vi "Bodies_GetPtInXYZ0.vi"(8 "error in (no error)":errorcluster, 10 "Point":T1, 11 "Bodies.lvclass":refnum<class "Bodies.lvclass">) -> (0 "error out":errorcluster, 1 "Coord4InGCS":T1={"Coord4"=[0.0, 0.0, 0.0, 1.0], "ID"=0}, 2 "PointInGCS":dbl[](array[numeric]) format="%#.6f", 3 "Bodies.lvclass 2":refnum<class "Bodies.lvclass">)   [LabVIEW 2015, in "Bodies.lvclass"]
uses:
  Bodies.lvclass
  PointOnBody.ctl
  Bodies.lvclass/Bodies.ctl
  <vilib>/Analysis/Matrix/Numeric/Conversions/Array To Matrix - RA2.vi
  <vilib>/Analysis/BLAS.llb/dgemv - General Matrix-Vector Product (DBL).vi
  <vilib>/Analysis/NI_AALBLAS.lvlib
  <vilib>/Analysis/Matrix/NI_Matrix.lvlib
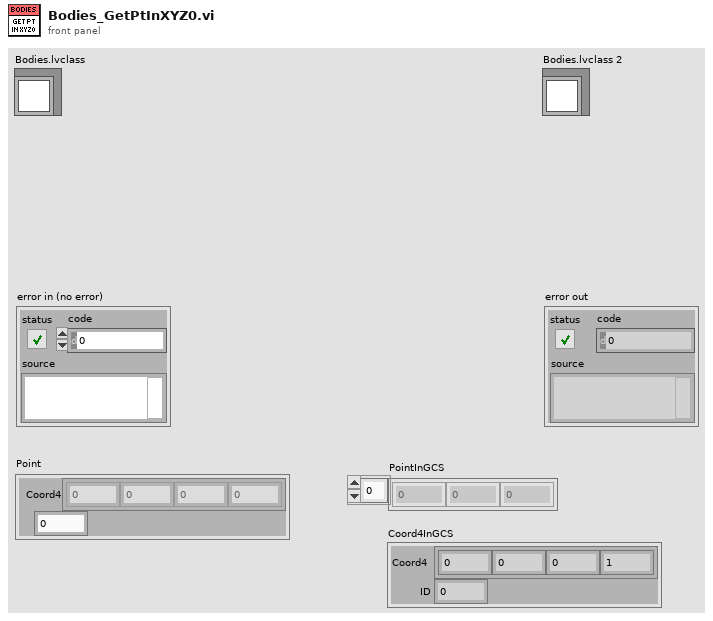
[diagram p1: front panel]
types:
  T1 = typedef "Bodies.lvclass/PointOnBody.ctl" = cluster{"Coord4":dbl[], "ID":i32}
  T2 = typedef "NI_Matrix.lvlib/RealMatrix.ctl" = dbl[][]
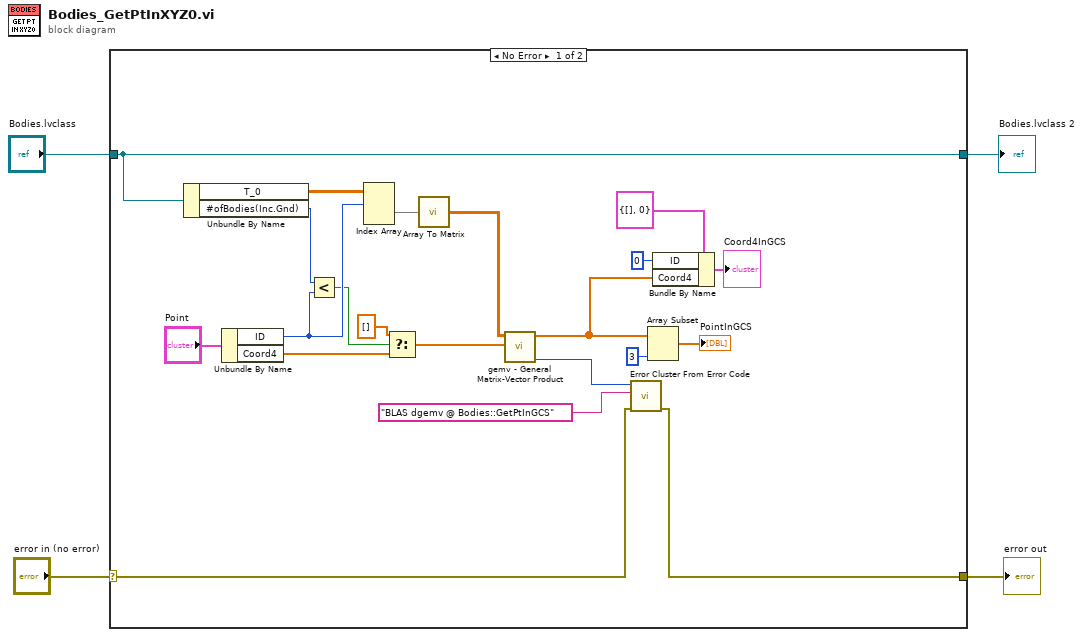
[diagram p0: block diagram]
diagram:
  n1 = case shown="No Error" "error in (no error)" {
    selector: "error in (no error)" -> [w19 w27]
    tunnel: "Bodies.lvclass" -> [w17 w26]
    tunnel: [w24 w27] -> w3
    tunnel: [w17 w26] -> w1
    frame No Error {
      n2 = Unbundle By Name(w17) -> ("T_0"=w16:dbl[][][], "#ofBodies(Inc.Gnd)"=w14:i32)
      n3 = Unbundle By Name("Point") -> ("ID"=w13:i32, "Coord4"=w11:dbl[])
      n4 = Less?(x=w14, y=w13) -> (x < y?=w12:bool)
      n5 = Index Array(array=w16, index (dim 0)=w13) -> (element=w18:dbl[][])  [unwired: 2 in]
      n6 = Select(t=dbl[] [], s=w12, f=w11) -> (s? t:f=w10:dbl[])
      n7 = call-poly <vilib>:"Array To Matrix.vi"("Real 2D Array"=w18) -> ("Real Matrix"=w15:T2)
      n8 = call-poly <vilib>:"gemv - General Matrix-Vector Product.vi"("x"=w10, "A"=w15) -> ("error"=w22:i32, "dgemv"=w8:dbl[])  [unwired: 8 in]
      n9 = call <vilib>:"Error Cluster From Error Code.vi"("error in (no error)"=w19, "error message (\"\")"="BLAS dgemv @ Bodies::GetPtInGCS" ("error source (\" \")"), "error code (0)"=w22) -> ("error out"=w24:errorcluster)  [unwired: 6 in]
      n10 = Array Subset(array=w8, length=3) -> (→"PointInGCS":dbl[])  [unwired: 1 in]
      n11 = Bundle By Name(cluster=T1 {"Coord4"=[], "ID"=0} ("Point 2"), "ID"=0, "Coord4"=w8) -> (→"Coord4InGCS":T1)
    }
    frame Error {
    }
  }
  "error out" <- w3
  "Bodies.lvclass 2" <- w1
